vi "Tosca-Setup Analog Input.vi"(0 "AI in":T2) -> (4 "AI out":T2, 8 "Canceled?":bool)   [LabVIEW 2020]
uses:
  Typedefs/Tosca-AI.ctl
  epl-vi-lib/Utility VIs/Buttons/KCheckmarkBoolean 2.ctl
  Sub VIs/Tosca-Globals.vi
panel:
  in  "Analog":i32(listbox)
  in  "Fs":dbl caption="Sampling rate (Hz)"
  in  "active":T1 caption="Active"
  out "exit signal":bool
  in  "Cancel":bool
  in  "OK":bool
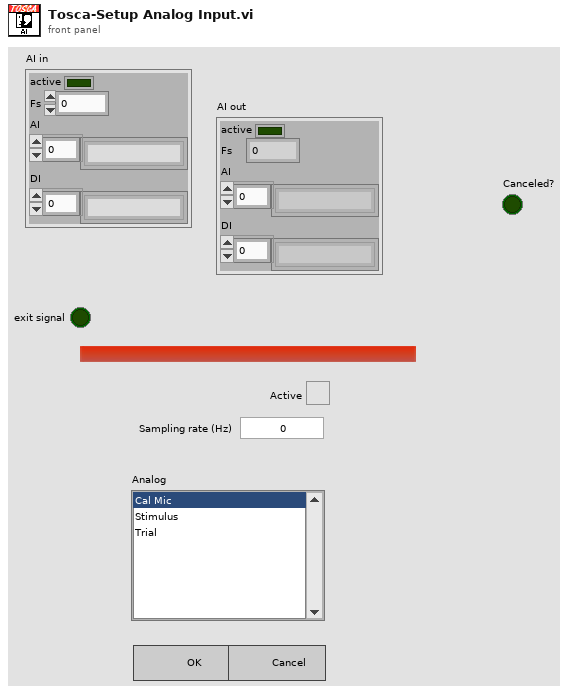
[diagram p1: front panel]
types:
  T1 = typedef "KCheckmarkBoolean 2.ctl" = bool
  T2 = typedef "Tosca-AI.ctl" = cluster{"active":bool, "Fs":dbl, "AI":string[], "DI":string[]}
  T3 = typedef "CM-Endpoint.ctl" = cluster{"Name":string, "Device":string}
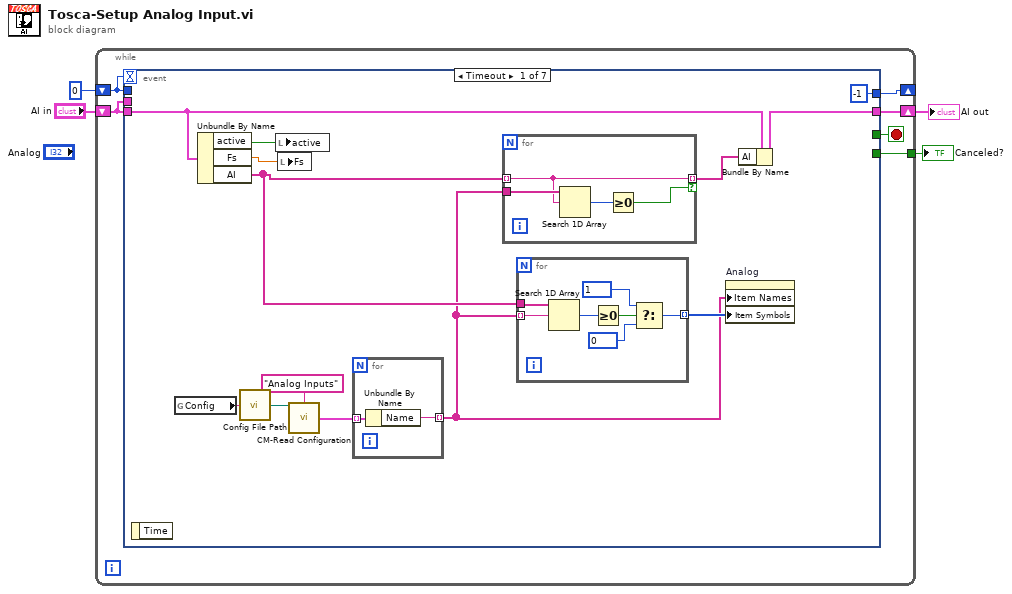
[diagram p0: block diagram]
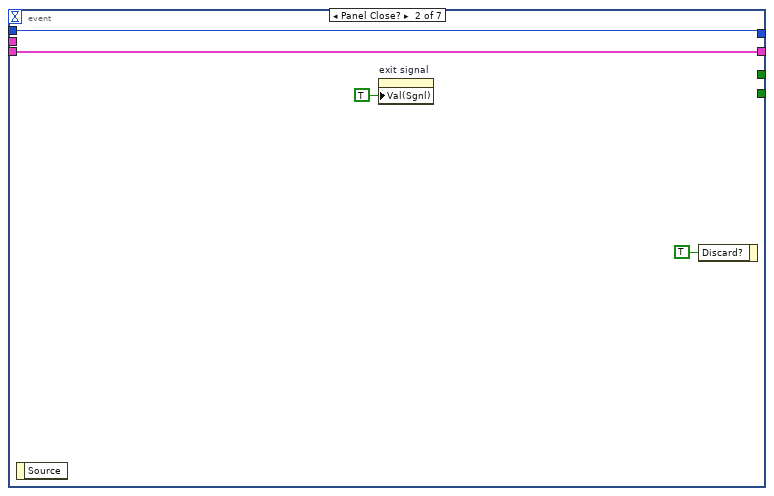
[diagram p2: hidden frame]
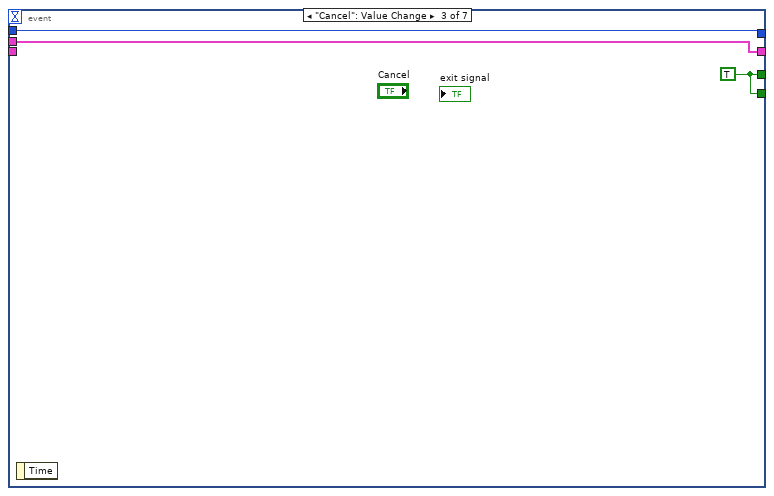
[diagram p3: hidden frame]
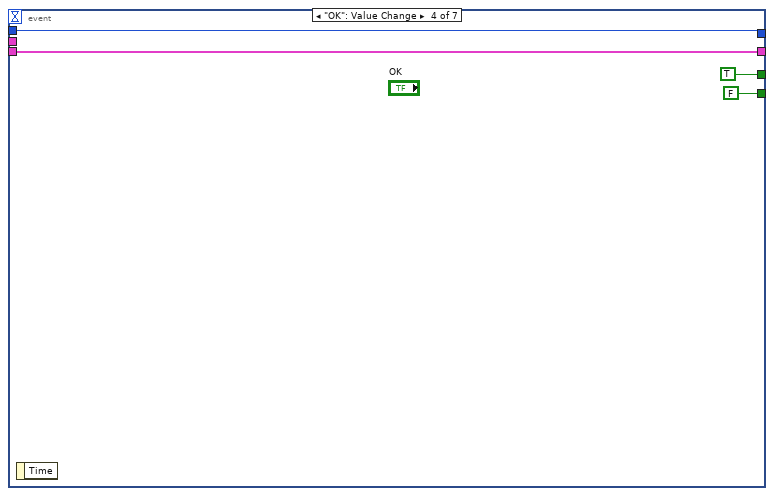
[diagram p4: hidden frame]
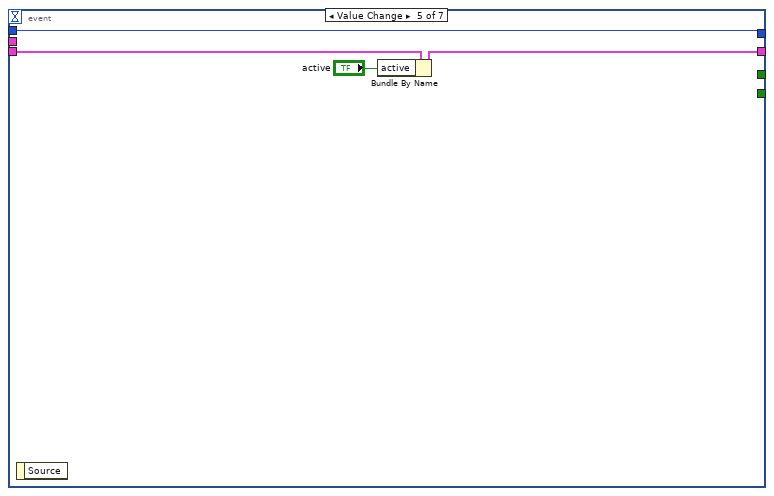
[diagram p5: hidden frame]
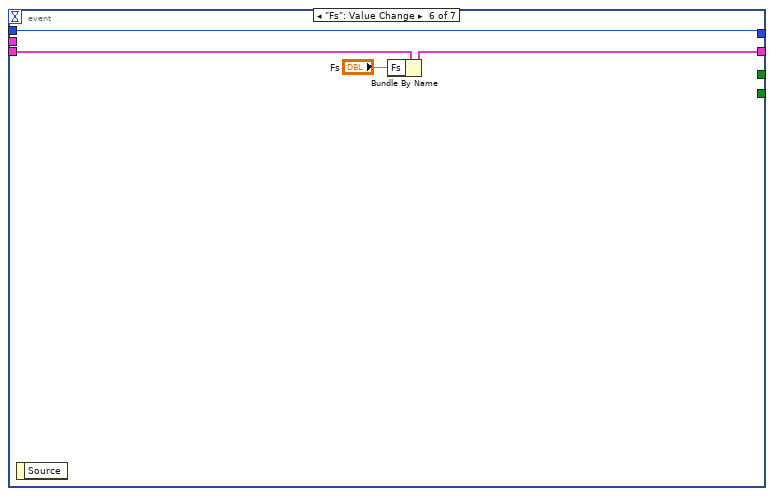
[diagram p6: hidden frame]
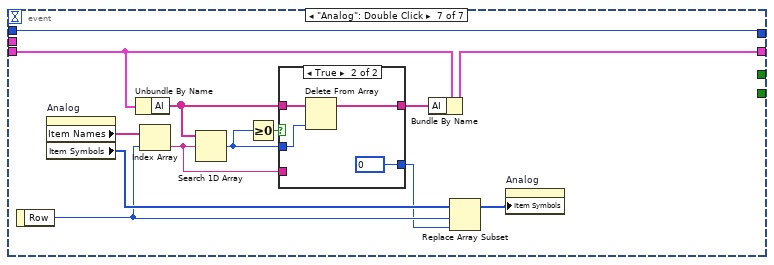
[diagram p7: hidden frame]
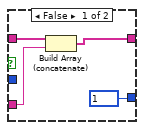
[diagram p8: hidden frame]
diagram:
  n1 = while {
    shift-right: [w10] -> _
    shift-left: 0 -> [w5]
    tunnel: [w7] -> w1
    shift-right: [w9] -> w2
    shift-left: "AI in" -> [w6]
    stop <- w8 stop-if-true
    n2 = event shown="[0] Timeout" {
      selector: _ -> [_ _ _ _ _ _ _]
      dyn-events: _ -> [_ _ _ _ _ _ _]
      timeout: w5 -> [_ _ _ _ _ _ _]
      tunnel: [-1 w40 w41 w44 w51 w55 w68] -> w10
      tunnel: w6 -> [w22 w39 _ w47 w50 w54 w66]
      tunnel: [w14 w39 w42 w47 w49 w53 w62] -> w9
      tunnel: [_ _ w43 TRUE _ _ _] -> w8
      tunnel: [_ _ w43 FALSE _ _ _] -> w7
      tunnel: w6 -> [_ _ w42 _ _ _ _]
      tunnel: w5 -> [_ w40 w41 w44 w51 w55 w68]
      event Timeout {
        n3 = event-data() -> ()  [unwired: 1 in, 1 out]
        n4 = global read "Tosca-Globals.vi" "Config"() -> (w18:string)
        n5 = Unbundle By Name(w22) -> ("active"=w21:bool, "Fs"=w20:dbl, "AI"=w12:string[])
        n6 = call "Config File Path.vi"("AppName"=w18) -> ("Default config file name"=w16:path)
        n7 = local write "active"(w21) -> ()
        n8 = local write "Fs"(w20) -> ()
        n9 = call "CM-Read Configuration.vi"("Connection File Path"=w16, "Section"="Analog Inputs") -> ("Endpoints"=w15:T3[])  [unwired: 9 in, 4 out]
        n10 = for {
          tunnel: w15 -> [w28] mode=indexing
          tunnel: [w29] -> w11 mode=indexing
          n11 = Unbundle By Name(w28) -> ("Name"=w29:string)
        }
        n12 = for {
          tunnel: [w26] -> w13 mode=indexing if=w24
          tunnel: w12 -> [w26] mode=indexing
          tunnel: w11 -> [w27]
          n13 = Search 1D Array(1D array=w27, element=w26) -> (index of element=w25:i32)  [unwired: 1 in]
          n14 = Greater Or Equal To 0?(x=w25) -> (x >= 0?=w24:bool)
        }
        n15 = for {
          tunnel: w11 -> [w35] mode=indexing
          tunnel: w12 -> [w36]
          tunnel: [w30] -> w19 mode=indexing
          n16 = Search 1D Array(1D array=w36, element=w35) -> (index of element=w34:i32)  [unwired: 1 in]
          n17 = Greater Or Equal To 0?(x=w34) -> (x >= 0?=w33:bool)
          n18 = Select(t=1, s=w33, f=0) -> (s? t:f=w30:i32)
        }
        n19 = property on="Analog" class="LstBox (strict)"("Item Names"=w11, "Item Symbols"=w19) -> ()  [unwired: 2 in, 2 out]
        n20 = Bundle By Name(cluster=w22, "AI"=w13) -> (w14:T2)
      }
      event Panel Close? {
        n21 = event-data() -> ()  [unwired: 1 in, 1 out]
        n22 = property on="exit signal" class="Bool (strict)"("Val(Sgnl)"=TRUE ("Value (Signaling)")) -> ()  [unwired: 2 in, 2 out]
        n23 = event-data("Discard?"=TRUE) -> ()  [unwired: 1 in, 1 out]
      }
      event "Cancel": Value Change {
        w43 = TRUE
        n24 = event-data() -> ()  [unwired: 1 in, 1 out]
      }
      event "OK": Value Change {
        n25 = event-data() -> ()  [unwired: 1 in, 1 out]
      }
      event Value Change {
        n26 = event-data() -> ()  [unwired: 1 in, 1 out]
        n27 = Bundle By Name(cluster=w50, "active"="active") -> (w49:T2)
      }
      event "Fs": Value Change {
        n28 = event-data() -> ()  [unwired: 1 in, 1 out]
        n29 = Bundle By Name(cluster=w54, "Fs"="Fs") -> (w53:T2)
      }
      event "Analog": Double Click {
        n30 = event-data() -> ("Row"=w58:i32)  [unwired: 1 in]
        n31 = property on="Analog" class="LstBox (strict)"() -> ("Item Names"=w67:string[], "Item Symbols"=w59:i32[])  [unwired: 2 in, 2 out]
        n32 = Unbundle By Name(w66) -> ("AI"=w63:string[])
        n33 = Index Array(array=w67, index=w58) -> (element=w60:string)
        n34 = Search 1D Array(1D array=w63, element=w60) -> (index of element=w65:i32)  [unwired: 1 in]
        n35 = Greater Or Equal To 0?(x=w65) -> (x >= 0?=w64:bool)
        n36 = case shown="True" w64 {
          tunnel: w65 -> [_ w76]
          tunnel: w63 -> [w72 w75]
          tunnel: [w71 w74] -> w61
          tunnel: w60 -> [w70 _]
          tunnel: [1 0] -> w56
          frame False {
            n37 = Build Array (concatenate)(w72, w70) -> (w71:string[])
          }
          frame True {
            n38 = Delete From Array(array=w75, index=w76) -> (array with subset deleted=w74:string[])  [unwired: 1 in, 1 out]
          }
        }
        n39 = Bundle By Name(cluster=w66, "AI"=w61) -> (w62:T2)
        n40 = Replace Array Subset(array=w59, new element=w56, index=w58) -> (w57:i32[])
        n41 = property on="Analog" class="LstBox (strict)"("Item Symbols"=w57) -> ()  [unwired: 2 in, 2 out]
      }
    }
  }
  "AI out" <- w2
  "Canceled?" <- w1
